vi "TimerUtil.vi"(10 "time (msec)":u32, 11 "typeTimer":u16(ring) items=["wait", "waitRandom"]) -> ()   [LabVIEW 2010]
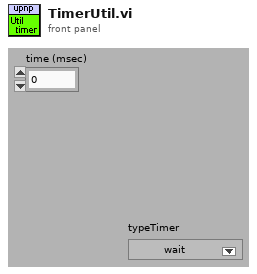
[diagram p1: front panel]
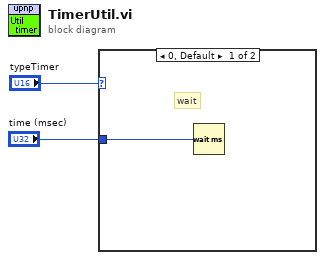
[diagram p0: block diagram]
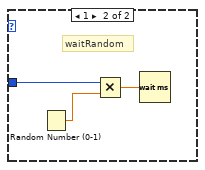
[diagram p2: hidden frame]
diagram:
  n1 = case shown="0, Default" "typeTimer" {
    tunnel: "time (msec)" -> [w3 w6]
    frame 0, Default {
      # "wait"
      n2 = Wait (ms)(milliseconds to wait=w3) -> ()  [unwired: 1 out]
    }
    frame 1 {
      # "waitRandom"
      n3 = Random Number (0-1)() -> (number: 0 to 1=w5:dbl)
      n4 = Multiply(x=w6, y=w5) -> (x*y=w4:dbl)
      n5 = Wait (ms)(milliseconds to wait=w4) -> ()  [unwired: 1 out]
    }
  }
